vi "Move For Time.vi"(8 "error in (no error)":errorcluster, 9 "Time (ms)":u32, 10 "Speed":dbl, 11 "intake.lvclass":refnum<class "intake.lvclass">) -> (0 "error out":errorcluster, 3 "intake.lvclass":refnum<class "intake.lvclass">)   [LabVIEW 2015, in "intake.lvclass"]
uses:
  intake.lvclass
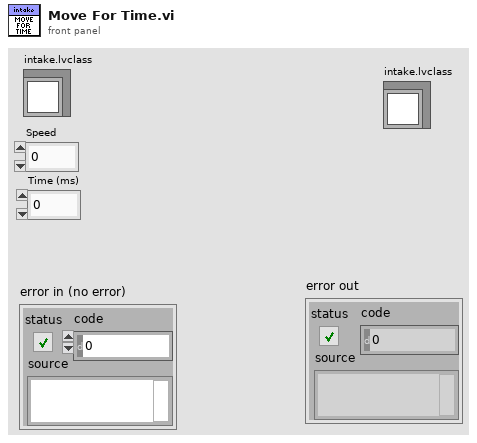
[diagram p1: front panel]
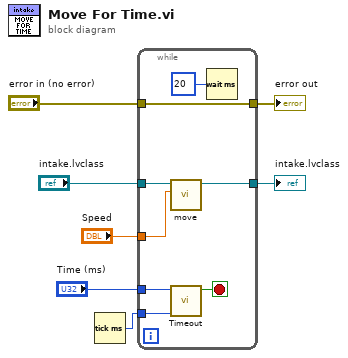
[diagram p0: block diagram]
diagram:
  n1 = Tick Count (ms)() -> (millisecond timer value=w5:u32)
  n2 = while {
    tunnel: [w12] -> w2
    tunnel: w5 -> [w14]
    tunnel: "Speed" -> [w9]
    tunnel: "Time (ms)" -> [w11]
    tunnel: "error in (no error)" -> [w10]
    tunnel: [w10] -> w3
    tunnel: "intake.lvclass" -> [w8]
    stop <- w13 stop-if-true
    n3 = call "move.vi"("Speed"=w9, "intake.lvclass"=w8) -> ("intake.lvclass"=w12:refnum<class "intake.lvclass">)  [unwired: 9 in]
    n4 = call "Timeout.vi"("Start Time In"=w14, "Time Limit"=w11) -> ("Timeout"=w13:bool)  [unwired: 8 in, 1 out]
    n5 = Wait (ms)(milliseconds to wait=u32 20) -> ()  [unwired: 1 out]
  }
  "error out" <- w3
  "intake.lvclass" <- w2
